vi "listDevsAndPorts.vi"() -> (2 "All Available Ports":string[](array[string]))   [LabVIEW 2022 SP3]
uses:
  <vilib>/Instr/_visa.llb/VISA Find Search Mode.ctl
  Globals/Meas_global.vi
  <resource>/objmgr/daqmx.rc
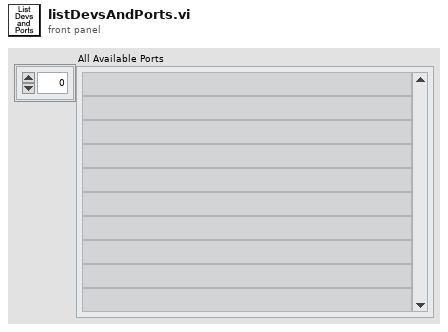
[diagram p1: front panel]
types:
  T1 = typedef "Post_Process.ctl" = enum16{"Take New Data", "Post Process Raw Data File"}
  T2 = typedef "VISA Find Search Mode.ctl" = u32
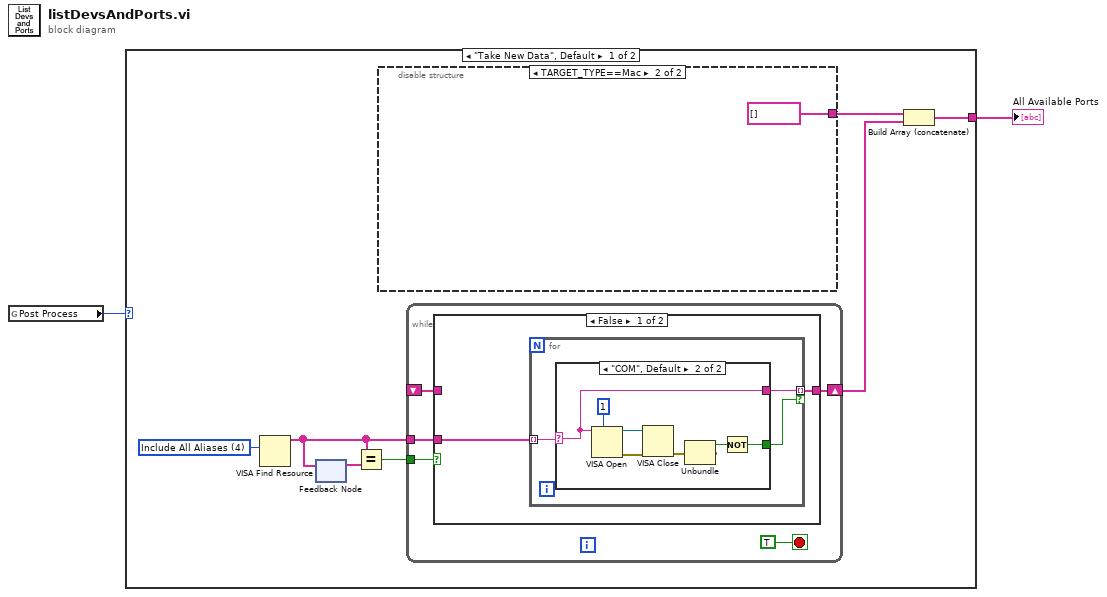
[diagram p0: block diagram]
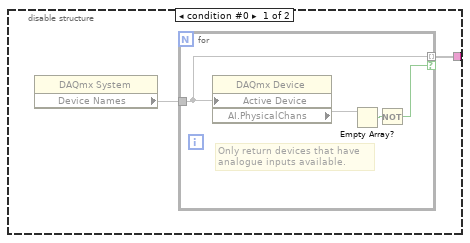
[diagram p2: hidden frame]
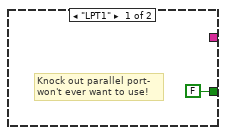
[diagram p3: hidden frame]
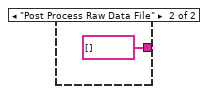
[diagram p5: hidden frame]
diagram:
  n1 = global read "Meas_global.vi" "Post Process"() -> (w1:T1)
  n2 = case shown="\"Take New Data\", Default" w1 {
    tunnel: [w3 string[] []] -> w2
    frame "Take New Data", Default {
      w9 = T2 4 items=["Canonical Names Only"=0, "Aliases Only"=2, "Include Matching Aliases"=3, "Include All Aliases"=4] ("Search Mode")
      n3 = VISA Find Resource(10:w9) -> (3:w7:string[])  [unwired: 2 in, 2 out]
      n4 = feedback #1() -> (w6:string[])  [unwired: 1 in]
      n5 = feedback-in #1(w7) -> ()
      n6 = Equal?(x=w7, y=w6) -> (x = y?=w4:bool)
      n7 = disable-structure shown="TARGET_TYPE==Mac" {
        disable-tunnel: [w10 string[] []] -> w8
        frame condition #0 {
          n8 = property class="DAQmx System"() -> ("Device Names"=w11)  [unwired: 2 in, 2 out]
          n9 = for {
            tunnel: w11 -> [w14]
            tunnel: [w14] -> w10 mode=indexing if=w12
            # "Only return devices that have\nanalogue inputs available."
            n10 = property class="DAQmx Device"("Active Device"=w14) -> ("AI.PhysicalChans"=w15)  [unwired: 2 in, 2 out]
            n11 = Empty Array?(array=w15) -> (empty?=w13:bool)
            n12 = Not(x=w13) -> (.not. x?=w12:bool)
          }
        }
        frame condition #1 (active) {
        }
      }
      n13 = while {
        tunnel: w7 -> [w21]
        shift-right: [w19] -> w5
        shift-left: _ -> [w17]
        tunnel: w4 -> [w18]
        stop <- TRUE stop-if-true
        n14 = case shown="False" w18 {
          tunnel: w21 -> [w23 _]
          tunnel: [w22 w35] -> w19
          tunnel: w17 -> [_ w35]
          frame False {
            n15 = for {
              tunnel: w23 -> [w26] mode=indexing
              tunnel: [w25] -> w22 mode=indexing if=w24
              n16 = case shown="\"COM\", Default" w26 {
                selector: w26 -> [_ w28]
                tunnel: [FALSE w30] -> w24
                tunnel: [_ w28] -> w25
                frame "LPT1" {
                  # "Knock out parallel port-\nwon't ever want to use!"
                }
                frame "COM", Default {
                  n17 = VISA Open(timeout (0)=u32 1 ("VISA Open timeout (0)"), VISA resource name=w28) -> (VISA resource name=w34:refnum<visa-resource-name>, error out=w33:errorcluster)  [unwired: 3 in]
                  n18 = VISA Close(VISA resource name=w34, error in (no error)=w33) -> (error out=w32:errorcluster)
                  n19 = Unbundle(w32) -> ("status"=w31:bool)  [unwired: 2 out]
                  n20 = Not(x=w31) -> (.not. x?=w30:bool)
                }
              }
            }
          }
          frame True {
          }
        }
      }
      n21 = Build Array (concatenate)(w8, w5) -> (w3:string[])
    }
    frame "Post Process Raw Data File" {
    }
  }
  "All Available Ports" <- w2
